vi "dpSubvi.vi"(1 "Array":dbl[][](array[numeric])) -> (0 "output array":dbl[][](array[numeric]))   [LabVIEW 2021]
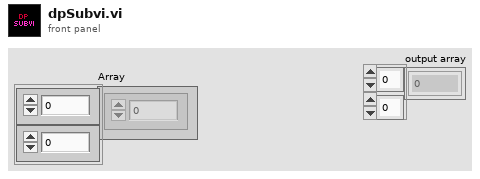
[diagram p1: front panel]
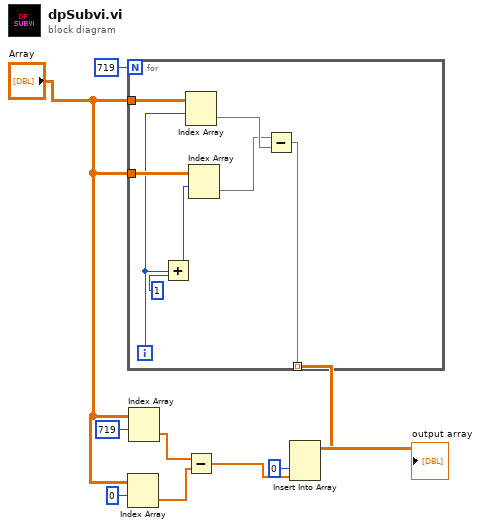
[diagram p0: block diagram]
diagram:
  n1 = for {
    N: 719 -> [_]
    tunnel: "Array" -> [w18]
    tunnel: "Array" -> [w17]
    tunnel: [w11] -> w1 mode=indexing
    i -> [w16]
    n2 = Add(x=w16, y=1) -> (x+y=w14:i32)
    n3 = Index Array "Index Array"(array=w18, index (row)=w16) -> (element=w13:dbl[])  [unwired: 1 in]
    n4 = Index Array "Index Array"(array=w17, index (row)=w14) -> (element=w12:dbl[])  [unwired: 1 in]
    n5 = Subtract(x=w12, y=w13) -> (x-y=w11:dbl[])
  }
  n6 = Index Array "Index Array"(array="Array", index (row)=0) -> (element=w6:dbl[])  [unwired: 1 in]
  n7 = Index Array "Index Array"(array="Array", index (row)=719) -> (element=w7:dbl[])  [unwired: 1 in]
  n8 = Subtract(x=w7, y=w6) -> (x-y=w3:dbl[])
  n9 = Insert Into Array "Insert Into Array"(array=w1, index (col)=0 ("disabled index (row)"), new element=w3) -> (→"output array":dbl[][])  [unwired: 1 in]
